vi "expt overnight automator 101freqs RT.vi"() -> ()   [LabVIEW 2018]
panel:
  in  "Save?":bool=TRUE
  in  "Field (Gauss)":u16(ring)=1 items=["9G"=1, "14G"=2]
  out "num coil iters done":i32
  out "total pos sweeps":i32
  out "total neg sweeps":i32
  in  "?":bool
  out "numSweeps list":i64[](array[numeric])=[10, 20, 10, 10, 20, 10]
  out "polarity list":i64[](array[numeric])=[-1, 1, -1, 1, -1, 1]
  in  "polarity pattern file":path=path "H:/rogers_data/Allende/S2-1-70_NRM/FOV1/P.txt"
  in  "num coil iterations":i32=1
  out "freq list (Hz)":dbl[](array[numeric])
  out "+Z current out (mA)":dbl=-975.0
  out "+Y current out (mA)":dbl=-1500.0
  out "+X current out (mA)":dbl=-20.0
  out "-Z current out (mA)":dbl=-975.0
  out "-Y current out (mA)":dbl=-1500.0
  out "-X current out (mA)":dbl=-20.0
  out "header cluster":T1
  in  "filename (adds .mat)":string="run_"
  in  "path":path=path "H:/RT/test"
  out "coil polarity":bool=TRUE
  out "img data stack pos":dbl[][](array[numeric])
  in  "Height":i64(slide)=1200 min=0 max=1200 step=4 scale=0.0..1200.0
  in  "Width":i64(slide)=1920 min=0 max=1920 step=4 scale=0.0..1920.0
  out "img data stack neg":dbl[][](array[numeric])
  in  "freq range":T2(ring)=enum."Both ranges"
  out "num freqs\n(set by field)":i32(ring)=101 items=["51", "101"]
  # "Coil parameters"
  # "Coil polarity"
  # "ODMR parameters"
  # "File setup"
  # "Camera parameters"
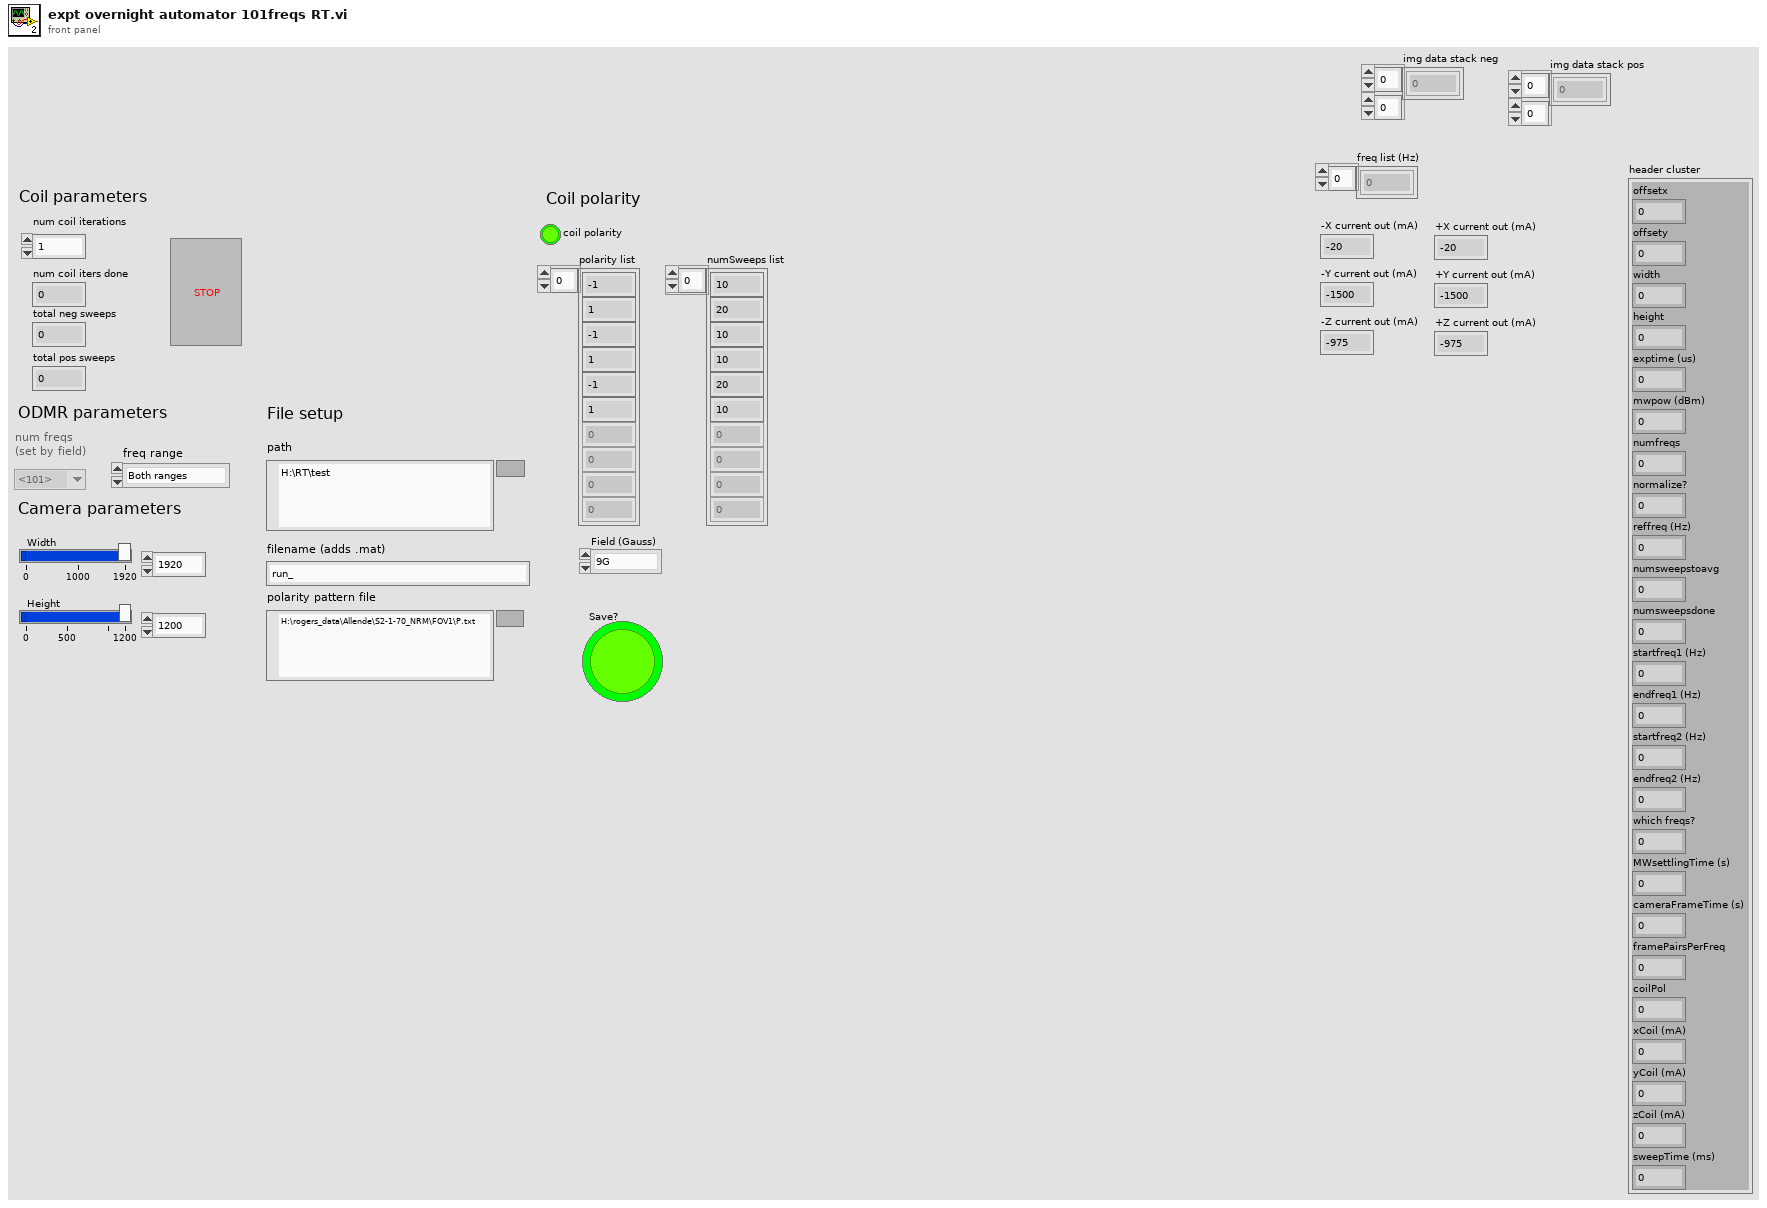
[diagram p1: front panel]
types:
  T1 = cluster{"offsetx":i64, "offsety":i64, "width":i64, "height":i64, "exptime (us)":dbl, "mwpow (dBm)":dbl, "numfreqs":i32, "normalize?":i32, "reffreq (Hz)":dbl, "numsweepstoavg":i32, "numsweepsdone":i32, "startfreq1 (Hz)":dbl, "endfreq1 (Hz)":dbl, "startfreq2 (Hz)":dbl, "endfreq2 (Hz)":dbl, "which freqs?":i32, "MWsettlingTime (s)":dbl, "cameraFrameTime (s)":dbl, "framePairsPerFreq":i32, "coilPol":i32, "xCoil (mA)":dbl, "yCoil (mA)":dbl, "zCoil (mA)":dbl, "sweepTime (ms)":i32}
  T2 = enum16{"Lower range", "Upper range", "Both ranges"}
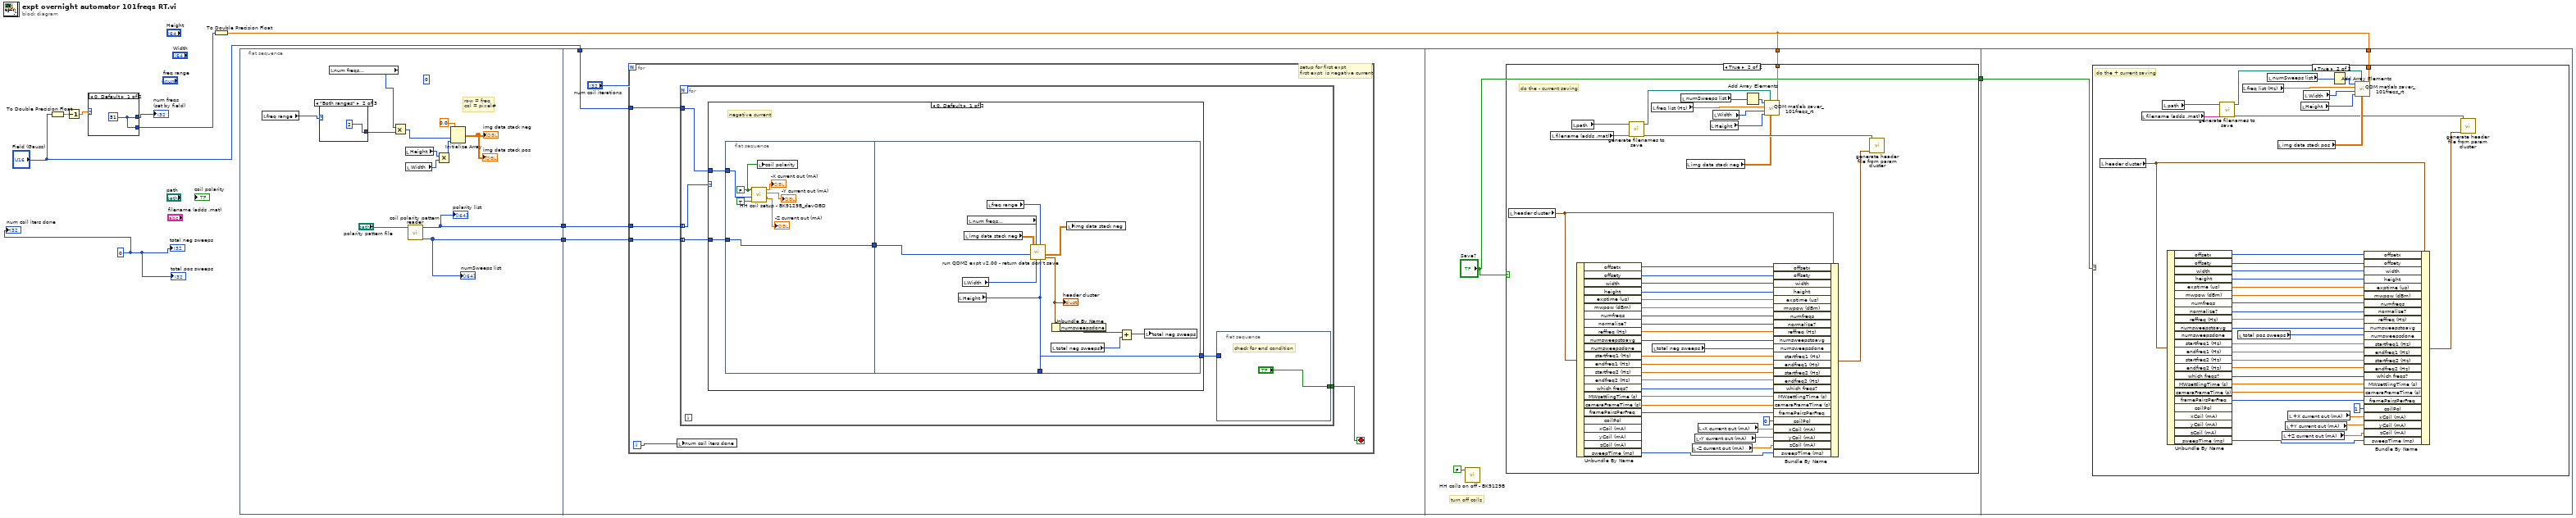
[diagram p0: block diagram]
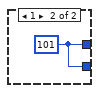
[diagram p2: hidden frame]
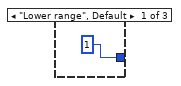
[diagram p3: hidden frame]
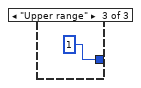
[diagram p4: hidden frame]
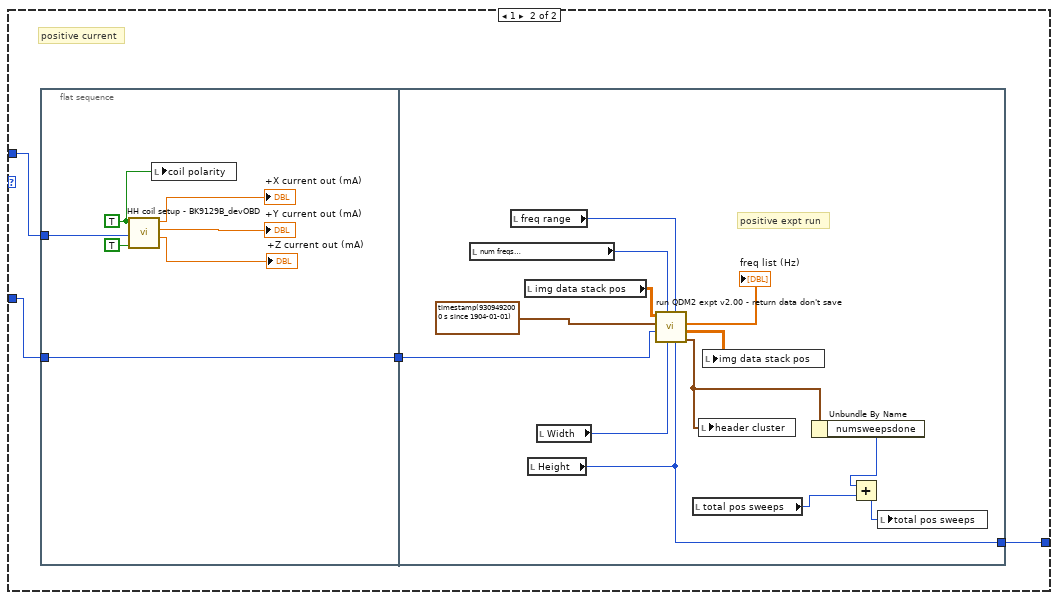
[diagram p5: hidden frame]
diagram:
  w8 = 0
  n1 = To Double Precision Float(number="Field (Gauss)") -> (double precision float=w4:dbl)
  n2 = Decrement(x=w4) -> (x-1=w3:dbl)
  n3 = case shown="0, Default" w3 {
    tunnel: [w11 w12] -> w5
    tunnel: [w11 w12] -> w2
    frame 0, Default {
      w11 = 51
    }
    frame 1 {
      w12 = 101
    }
  }
  "num freqs\n(set by field)" <- w5
  n4 = To Double Precision Float(number=w2) -> (double precision float=w1:dbl)
  n5 = flat-sequence {
    tunnel: [w14] -> w10
    tunnel: [w13] -> w9
    tunnel: w10 -> [w31]
    tunnel: w9 -> [w30]
    tunnel: "Field (Gauss)" -> [w28]
    tunnel: ["Save?"] -> w7
    tunnel: w1 -> [w89]
    tunnel: w7 -> [w130]
    tunnel: w1 -> [w129]
    frame #0 {
      (unwired) 0 ("1st half sweeps")
      # "row = freq\ncol = pixel#"
      n6 = local read "freq range"() -> (w16:T2)
      n7 = case shown="\"Both ranges\"" w16 {
        tunnel: [1 ("numFreqs") 2 ("numFreqs") 1 ("numFreqs")] -> w19
        frame "Lower range", Default {
        }
        frame "Both ranges" {
        }
        frame "Upper range" {
        }
      }
      n8 = local read "num freqs\n(set by field)"() -> (w17:i32)
      n9 = Multiply(x=w17, y=w19) -> (x*y=w18:i32)
      n10 = local read "Height"() -> (w24:i64)
      n11 = local read "Width"() -> (w23:i64)
      n12 = call "coil polarity pattern reader.vi"("polarity pattern file"="polarity pattern file") -> ("numSweeps list"=w13:i64[], "polarity list"=w14:i64[])  [unwired: 9 in]
      "polarity list" <- w14
      "numSweeps list" <- w13
      n13 = Multiply(x=w24, y=w23) -> (x*y=w22:i64)
      n14 = Initialize Array(0.0 ("element"), w18, w22) -> (→"img data stack pos" →"img data stack neg":dbl[][])
    }
    frame #1 {
      n15 = for {
        N: "num coil iterations" -> [_]
        tunnel: w31 -> [w36]
        tunnel: w30 -> [w35]
        tunnel: w28 -> [w32]
        i -> [w33]
        stop <- w34 stop-if-true
        # "setup for first expt\nfirst expt  is negative current"
        n16 = local write "num coil iters done"(w33) -> ()
        n17 = for {
          tunnel: w36 -> [w41] mode=indexing
          tunnel: w35 -> [w40] mode=indexing
          tunnel: [w38] -> w34
          tunnel: w32 -> [w37]
          n18 = case shown="0, Default" w41 {
            tunnel: w40 -> [w45 w68]
            tunnel: [w44 w66] -> w39
            tunnel: w37 -> [w43 w65]
            frame 0, Default {
              # "negative current"
              n19 = flat-sequence {
                tunnel: [w53] -> w46
                tunnel: w45 -> [w53]
                tunnel: w43 -> [w47]
                tunnel: w46 -> [w59]
                tunnel: [w58] -> w44
                frame #0 {
                  w52 = FALSE ("coil polarity")
                  n20 = call "HH coil setup - BK9129B_devOBD.VI"("setup enabled?"=TRUE, "number"=w47, "coil polarity"=w52) -> ("Z current out (mA)"=→"-Z current out (mA)":dbl, "Y current out (mA)"=→"-Y current out (mA)":dbl, "X current out (mA)"=→"-X current out (mA)":dbl)  [unwired: 6 in]
                  n21 = local write "coil polarity"(w52) -> ()
                }
                frame #1 {
                  n22 = local read "Height"() -> (w58:i64)
                  n23 = local read "Width"() -> (w62:i64)
                  n24 = local read "img data stack neg"() -> (w60:dbl[][])
                  n25 = local read "num freqs\n(set by field)"() -> (w64:i32)
                  n26 = local read "freq range"() -> (w63:T2)
                  n27 = call "run QDM2 expt v2.00 - return data don't save.vi"("Height"=w58, "which freqs?"=w63, "Width"=w62, "numFreqs"=w64, "num sweeps to avg"=w59, "img data stack Input"=w60) -> ("header cluster"=w57:T1, "img data stack Return"=w61:dbl[][])  [unwired: 2 in, 2 out]
                  "header cluster" <- w57
                  n28 = local read "total neg sweeps"() -> (w55:i32)
                  n29 = Unbundle By Name(w57) -> ("numsweepsdone"=w56:i32)
                  n30 = local write "img data stack neg"(w61) -> ()
                  n31 = Add(x=w56, y=w55) -> (x+y=w54:i32)
                  n32 = local write "total neg sweeps"(w54) -> ()
                }
              }
            }
            frame 1 {
              # "positive current"
              n33 = flat-sequence {
                tunnel: w68 -> [w70]
                tunnel: [w70] -> w67
                tunnel: w65 -> [w69]
                tunnel: w67 -> [w81]
                tunnel: [w80] -> w66
                frame #0 {
                  w71 = TRUE ("coil polarity")
                  n34 = call "HH coil setup - BK9129B_devOBD.VI"("setup enabled?"=TRUE, "number"=w69, "coil polarity"=w71) -> ("Z current out (mA)"=→"+Z current out (mA)":dbl, "Y current out (mA)"=→"+Y current out (mA)":dbl, "X current out (mA)"=→"+X current out (mA)":dbl)  [unwired: 6 in]
                  n35 = local write "coil polarity"(w71) -> ()
                }
                frame #1 {
                  # "positive expt run"
                  n36 = local read "num freqs\n(set by field)"() -> (w88:i32)
                  n37 = local read "freq range"() -> (w87:T2)
                  n38 = local read "img data stack pos"() -> (w83:dbl[][])
                  n39 = local read "Height"() -> (w80:i64)
                  n40 = local read "Width"() -> (w86:i64)
                  n41 = call "run QDM2 expt v2.00 - return data don't save.vi"("Height"=w80, "which freqs?"=w87, "Width"=w86, "numFreqs"=w88, "num sweeps to avg"=w81, 10:timestamp(9309492000 s since 1904-01-01) ("cutoff time"), "img data stack Input"=w83) -> ("header cluster"=w79:T1, "img data stack Return"=w84:dbl[][], "freq list (Hz)"=→"freq list (Hz)":dbl[])  [unwired: 1 in, 1 out]
                  n42 = local read "total pos sweeps"() -> (w77:i32)
                  n43 = local write "header cluster"(w79) -> ()
                  n44 = local write "img data stack pos"(w84) -> ()
                  n45 = Unbundle By Name(w79) -> ("numsweepsdone"=w78:i32)
                  n46 = Add(x=w78, y=w77) -> (x+y=w76:i32)
                  n47 = local write "total pos sweeps"(w76) -> ()
                }
              }
            }
          }
          n48 = flat-sequence {
            tunnel: w39 -> [_]
            tunnel: ["?"] -> w38
            frame #0 {
              # "check for end condition"
            }
          }
        }
      }
    }
    frame #2 {
      # "turn off coils"
      n49 = call "HH coils on off - BK9129B.VI"("coils on?"=FALSE) -> ()  [unwired: 11 in]
      n50 = case shown="True" "Save?" {
        tunnel: w89 -> [_ w92]
        frame False {
        }
        frame True {
          # "do the - current saving"
          n51 = local read "header cluster"() -> (w103:T1)
          n52 = local read "filename (adds .mat)"() -> (w127:string)
          n53 = local read "path"() -> (w128:path)
          n54 = Unbundle By Name(w103) -> ("offsetx"=w104:i64, "offsety"=w105:i64, "width"=w106:i64, "height"=w107:i64, "exptime (us)"=w108:dbl, "mwpow (dBm)"=w109:dbl, "numfreqs"=w110:i32, "normalize?"=w111:i32, "reffreq (Hz)"=w112:dbl, "numsweepstoavg"=w113:i32, "startfreq1 (Hz)"=w114:dbl, "endfreq1 (Hz)"=w115:dbl, "startfreq2 (Hz)"=w116:dbl, "endfreq2 (Hz)"=w117:dbl, "which freqs?"=w118:i32, "MWsettlingTime (s)"=w119:dbl, "cameraFrameTime (s)"=w120:dbl, "framePairsPerFreq"=w121:i32, "sweepTime (ms)"=w122:i32)  [unwired: 5 out]
          n55 = call "generate filenames to save.vi"("filename (adds .mat)"=w127, "path"=w128) -> ("header path"=w126:path, "matlab path"=w101:path)  [unwired: 8 in]
          n56 = local read "freq list (Hz)"() -> (w97:dbl[])
          n57 = local read "total neg sweeps"() -> (w93:i32)
          n58 = local read "numSweeps list"() -> (w95:i64[])
          n59 = local read "img data stack neg"() -> (w98:dbl[][])
          n60 = local read "-Z current out (mA)"() -> (w125:dbl)
          n61 = local read "-Y current out (mA)"() -> (w124:dbl)
          n62 = local read "-X current out (mA)"() -> (w123:dbl)
          n63 = local read "Height"() -> (w99:i64)
          n64 = local read "Width"() -> (w100:i64)
          n65 = Add Array Elements(numeric array=w95) -> (sum=w94:i64)
          n66 = call "QDM matlab saver_101freqs_rt.vi"("NumofFreq"=w92, "img data stack Input"=w98, "matlab path"=w101, "Height"=w99, "Width"=w100, "freq list (Hz)"=w97, "sweep #"=w94) -> ()  [unwired: 5 in]
          n67 = Bundle By Name(cluster=w103, "offsetx"=w104, "offsety"=w105, "width"=w106, "height"=w107, "exptime (us)"=w108, "mwpow (dBm)"=w109, "numfreqs"=w110, "normalize?"=w111, "reffreq (Hz)"=w112, "numsweepstoavg"=w113, "numsweepsdone"=w93, "startfreq1 (Hz)"=w114, "endfreq1 (Hz)"=w115, "startfreq2 (Hz)"=w116, "endfreq2 (Hz)"=w117, "which freqs?"=w118, "MWsettlingTime (s)"=w119, "cameraFrameTime (s)"=w120, "framePairsPerFreq"=w121, "coilPol"=0, "xCoil (mA)"=w123, "yCoil (mA)"=w124, "zCoil (mA)"=w125, "sweepTime (ms)"=w122) -> (w102:T1)
          n68 = call "generate header file from param cluster.vi"("output cluster"=w102, "header path (full)"=w126) -> ()  [unwired: 10 in]
        }
      }
    }
    frame #3 {
      n69 = case shown="True" w130 {
        tunnel: w129 -> [_ w131]
        frame False {
        }
        frame True {
          # "do the + current saving"
          n70 = local read "header cluster"() -> (w161:T1)
          n71 = local read "filename (adds .mat)"() -> (w137:string)
          n72 = local read "path"() -> (w136:path)
          n73 = Unbundle By Name(w161) -> ("offsetx"=w160:i64, "offsety"=w159:i64, "width"=w158:i64, "height"=w157:i64, "exptime (us)"=w156:dbl, "mwpow (dBm)"=w155:dbl, "numfreqs"=w154:i32, "normalize?"=w153:i32, "reffreq (Hz)"=w152:dbl, "numsweepstoavg"=w151:i32, "startfreq1 (Hz)"=w150:dbl, "endfreq1 (Hz)"=w149:dbl, "startfreq2 (Hz)"=w148:dbl, "endfreq2 (Hz)"=w147:dbl, "which freqs?"=w146:i32, "MWsettlingTime (s)"=w145:dbl, "cameraFrameTime (s)"=w144:dbl, "framePairsPerFreq"=w143:i32, "sweepTime (ms)"=w142:i32)  [unwired: 5 out]
          n74 = call "generate filenames to save.vi"("filename (adds .mat)"=w137, "path"=w136) -> ("header path"=w138:path, "matlab path"=w163:path)  [unwired: 8 in]
          n75 = local read "total pos sweeps"() -> (w132:i32)
          n76 = local read "freq list (Hz)"() -> (w167:dbl[])
          n77 = local read "numSweeps list"() -> (w134:i64[])
          n78 = local read "img data stack pos"() -> (w166:dbl[][])
          n79 = local read "+Z current out (mA)"() -> (w139:dbl)
          n80 = local read "+Y current out (mA)"() -> (w140:dbl)
          n81 = local read "+X current out (mA)"() -> (w141:dbl)
          n82 = local read "Height"() -> (w165:i64)
          n83 = local read "Width"() -> (w164:i64)
          n84 = Add Array Elements(numeric array=w134) -> (sum=w133:i64)
          n85 = call "QDM matlab saver_101freqs_rt.vi"("NumofFreq"=w131, "img data stack Input"=w166, "matlab path"=w163, "Height"=w165, "Width"=w164, "freq list (Hz)"=w167, "sweep #"=w133) -> ()  [unwired: 5 in]
          n86 = Bundle By Name(cluster=w161, "offsetx"=w160, "offsety"=w159, "width"=w158, "height"=w157, "exptime (us)"=w156, "mwpow (dBm)"=w155, "numfreqs"=w154, "normalize?"=w153, "reffreq (Hz)"=w152, "numsweepstoavg"=w151, "numsweepsdone"=w132, "startfreq1 (Hz)"=w150, "endfreq1 (Hz)"=w149, "startfreq2 (Hz)"=w148, "endfreq2 (Hz)"=w147, "which freqs?"=w146, "MWsettlingTime (s)"=w145, "cameraFrameTime (s)"=w144, "framePairsPerFreq"=w143, "coilPol"=1, "xCoil (mA)"=w141, "yCoil (mA)"=w140, "zCoil (mA)"=w139, "sweepTime (ms)"=w142) -> (w162:T1)
          n87 = call "generate header file from param cluster.vi"("output cluster"=w162, "header path (full)"=w138) -> ()  [unwired: 10 in]
        }
      }
    }
  }
  "total neg sweeps" <- w8
  "total pos sweeps" <- w8
  "num coil iters done" <- w8
